vi "Get Number Of Items.vi"(8 "error in (no error)":errorcluster, 11 "IContainer in":refnum<class "IContainer.lvclass">) -> (0 "error out":errorcluster, 2 "Items":i32, 3 "IContainer out":refnum<class "IContainer.lvclass">)   [LabVIEW 2013, in "IContainer.lvclass"]
doc: "Copyright 2018, Wiebe Walstra, wiebe@carya.nl."
uses:
  IContainer.lvclass
  IContainer.lvclass/IContainer.ctl
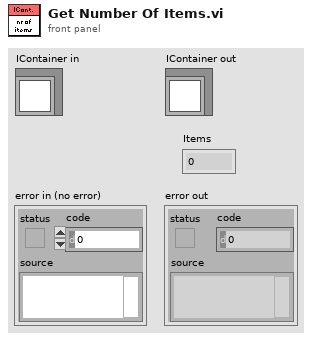
[diagram p1: front panel]
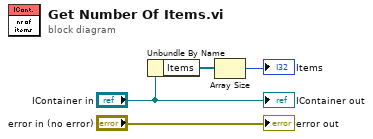
[diagram p0: block diagram]
diagram:
  n1 = Unbundle By Name("IContainer in") -> ("Items"=w2:refnum<class "IObject.lvclass">[])
  n2 = Array Size(array=w2) -> (size(s)=→"Items":i32)
  "error out" <- "error in (no error)"
  "IContainer out" <- "IContainer in"
